vi "Write Multiple Coils.vi"(8 "error in":errorcluster, 9 "coils to write":bool[](array[boolean]), 10 "starting address":u16, 11 "Modbus master in":refnum<class "Modbus Master.lvclass">) -> (0 "error out":errorcluster, 3 "Modbus master out":refnum<class "Modbus Master.lvclass">)   [LabVIEW 2015, in "Modbus Library.lvlib" / "Modbus Master.lvclass"]
doc: "Writes <B>coils to write</B> starting at <B>starting address</B> to the device coils."
uses:
  Modbus Master.lvclass
  Modbus Master.lvclass/Modbus Master.ctl
  Modbus API.lvclass/Modbus API.ctl
  Transmission Data Unit/Transmission Data Unit.lvclass
  Master Function Definition/Master Function Definition.lvclass
  Modbus API.lvclass
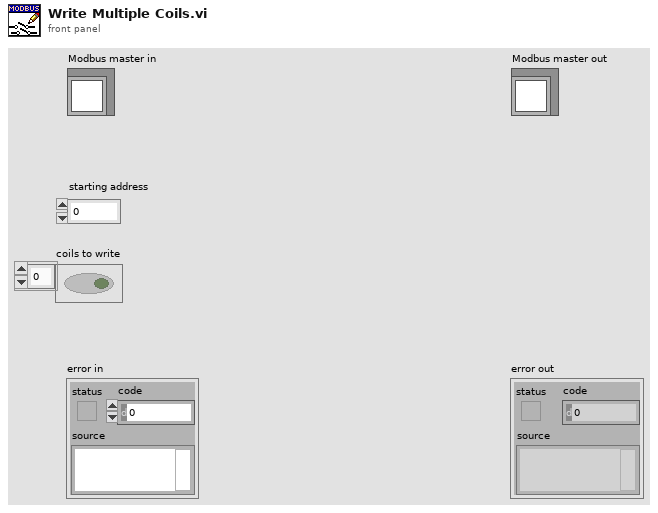
[diagram p1: front panel]
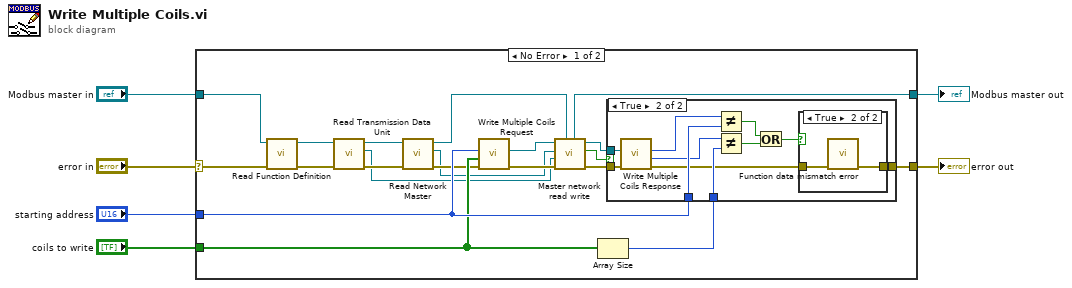
[diagram p0: block diagram]
diagram:
  n1 = case shown="No Error" "error in" {
    selector: "error in" -> [w13 w43]
    tunnel: "Modbus master in" -> [w8 w42]
    tunnel: [w25 w43] -> w5
    tunnel: [w18 w42] -> w6
    tunnel: "starting address" -> [w24 _]
    tunnel: "coils to write" -> [w23 _]
    frame No Error {
      n2 = call "Read Function Definition.vi"("error in"=w13, "Modbus master in"=w8) -> ("error out"=w15:errorcluster, "Modbus master out"=w16:refnum<class "Modbus Master.lvclass">)  [unwired: 7 in, 1 out]
      n3 = call "Read Transmission Data Unit.vi"("error in"=w15, "Modbus instance in"=w16) -> ("error out"=w14:errorcluster, "transmission data unit"=w9:refnum<class "Transmission Data Unit.lvclass">, "Modbus instance out"=w17:refnum<class "Modbus Master.lvclass">)  [unwired: 7 in]
      n4 = call "Read Network Master.vi"("error in"=w14, "Modbus master in"=w17) -> ("error out"=w12:errorcluster, "network master"=w10:refnum<class "Network Master.lvclass">, "Modbus master out"=w11:refnum<class "Modbus Master.lvclass">)  [unwired: 7 in]
      n5 = call "Write Multiple Coils Request.vi"("error in"=w12, "Coils To Write"=w23, "Starting Address"=w24) -> ("error out"=w26:errorcluster, "modbus data unit out"=w19:refnum<class "Modbus Data Unit.lvclass">)  [unwired: 7 in]
      n6 = call "Master network read write.vi"("Modbus master in"=w11, "error in"=w26, "transmission data unit in"=w9, "network master in"=w10, "Modbus data unit in"=w19) -> ("error out"=w21:errorcluster, "PDU Valid?"=w7:bool, "Modbus data unit out"=w20:refnum<class "Modbus Data Unit.lvclass">, "Modbus master out"=w18:refnum<class "Modbus Master.lvclass">)  [unwired: 3 in]
      n7 = Array Size(array=w23) -> (size(s)=w22:i32)
      n8 = case shown="True" w7 {
        tunnel: [w27 w35] -> w25
        tunnel: w24 -> [_ w33]
        tunnel: w22 -> [_ w31]
        tunnel: w21 -> [w27 w30]
        tunnel: w20 -> [_ w29]
        frame False {
        }
        frame True {
          n9 = call "Write Multiple Coils Response.vi"("error in"=w30, "modbus data unit in"=w29) -> ("error out"=w28:errorcluster, "Number of Coils"=w32:u16, "Start Address"=w34:u16)  [unwired: 7 in]
          n10 = Not Equal?(x=w34, y=w33) -> (x != y?=w37:bool)
          n11 = Not Equal?(x=w32, y=w31) -> (x != y?=w36:bool)
          n12 = Or(x=w37, y=w36) -> (x .or. y?=w38:bool)
          n13 = case shown="True" w38 {
            tunnel: [w39 w40] -> w35
            tunnel: w28 -> [w39 w41]
            frame False {
            }
            frame True {
              n14 = call "Function data mismatch error.vi"("error in (no error)"=w41) -> ("error out"=w40:errorcluster)  [unwired: 10 in]
            }
          }
        }
      }
    }
    frame Error {
    }
  }
  "error out" <- w5
  "Modbus master out" <- w6
